vi "Post Substeps Digital Input Task.vi"(9 "Socket No":u16=1, 10 "DI In":T1, 11 "Sequence Context In":refnum<k7>) -> (0 "error out":errorcluster, 1 "PhysicalChannel":string[](array[string]), 2 "DigitalInputRead":bool[](array[boolean]), 3 "Report Text":string)   [LabVIEW 2023, in "LTT_TeststandSteptypes.lvlib"]
doc: "This VI is Anaload Input Read MultiNumeric Test and PostSub Steptypes"
uses:
  LTT_TeststandSteptypes.lvlib
  HardwareAbstractionLayer_LVOOP/Digital Input/DI_class/DI DAQ/Control/DI Step Control.ctl
  HardwareAbstractionLayer_LVOOP/Main/Class Options.ctl
  HardwareAbstractionLayer_LVOOP/Digital Input/DI_class/DI.lvclass
  HardwareAbstractionLayer_LVOOP/Main/Main.lvclass
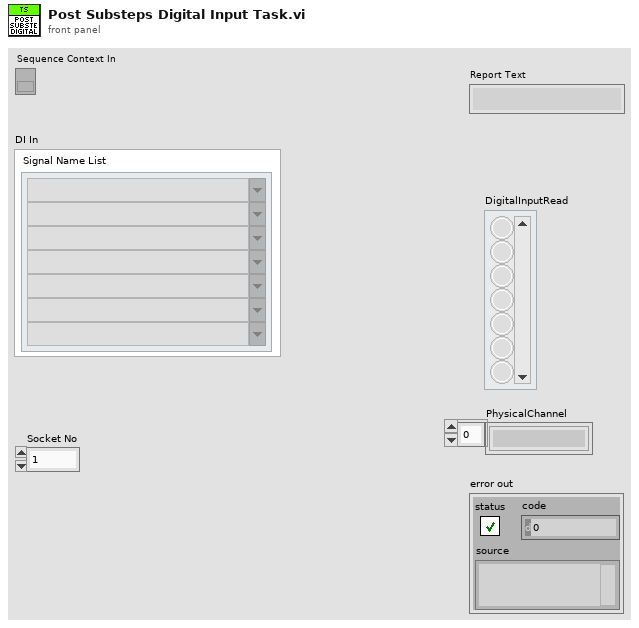
[diagram p1: front panel]
types:
  T1 = typedef "HardwareAbstractionLayer_LVOOP.lvlib/DI.lvclass/DI Step Control.ctl" = cluster{"Signal Name List":string[]}
  T2 = typedef "HardwareAbstractionLayer_LVOOP.lvlib/Main.lvclass/Class Options.ctl" = enum16{"Init All Class", "Read All Class", "Write AI Class", "Write AO Class", "Write AO Waveform Generation", "Write DI Class", "Write DO Class", "Write PWM Input Class", "Write PWM Output Class", "Exit"}
  T3 = typedef "HardwareAbstractionLayer_LVOOP.lvlib/Main.lvclass/Class Ref.ctl" = cluster{"FGV":refnum<class "Function Global Variable.lvclass">, "Notifier":refnum<class "NotifierHandler.lvclass">, "Queue":refnum<class "Queue Handler.lvclass">, "User Event":refnum<class "User Event.lvclass">, "Data Manager":refnum<class "Data Manager.lvclass">, "DMM":refnum<class "DMM.lvclass">, "Function Generator":refnum<class "Function Generator.lvclass">, "Oscilloscope":refnum<class "Oscilloscope.lvclass">, "PowerSupply":refnum<class "PowerSupply.lvclass">, "Teststand":refnum<class "Teststand.lvclass">, "AO":refnum<class "AO.lvclass">, "AI":refnum<class "AI.lvclass">, "Database":refnum<class "Database.lvclass">, "AO Waveform Generation":refnum<class "AO.lvclass">, "DO":refnum<class "DO.lvclass">, "DI":refnum<class "DI.lvclass">, "PWM Output":refnum<class "PWM Output.lvclass">, "PWM Input":refnum<class "PWM Input.lvclass">, "RelayOutput":refnum<class "NISwitch.lvclass">, "Modbus":refnum<class "Modbus.lvclass">, "CAN":refnum<class "CAN.lvclass">}
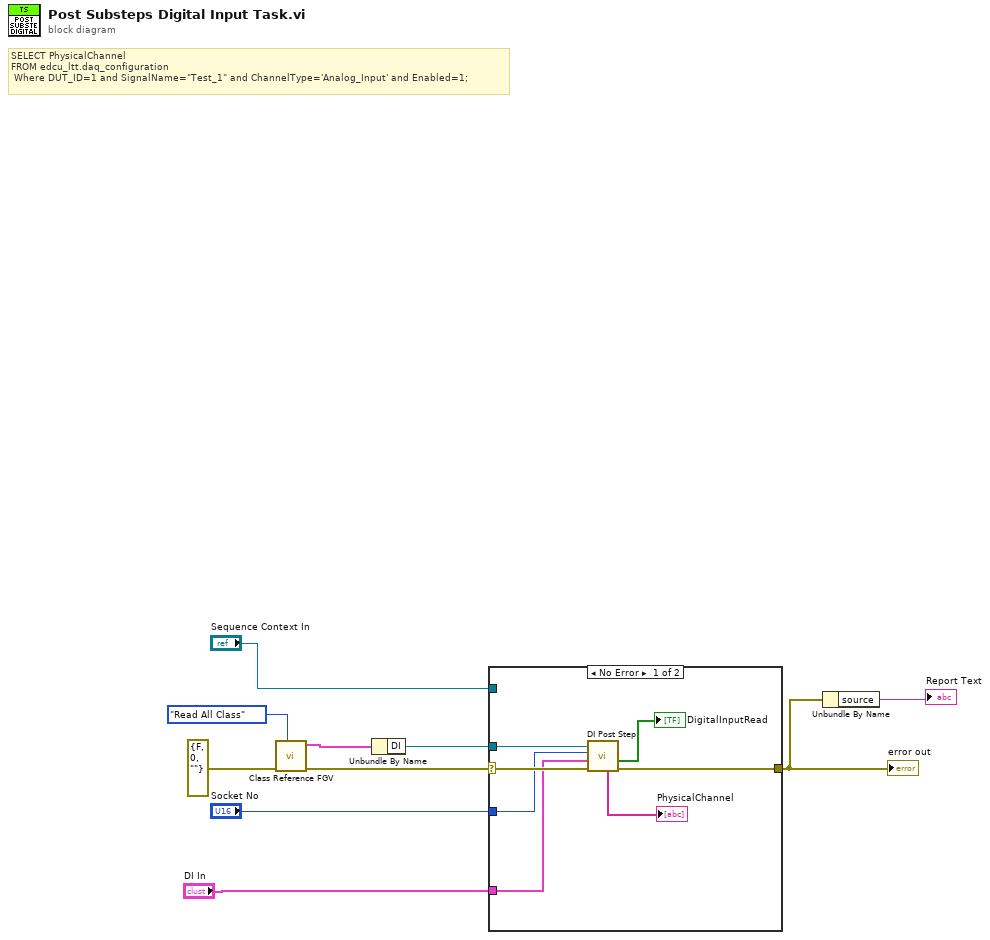
[diagram p0: block diagram]
diagram:
  # "SELECT PhysicalChannel \nFROM edcu_ltt.daq_configuration\n Where DUT_ID=1 and SignalName=\"Test_1\" and ChannelType='Analog_Input' and Enabled=1;"
  n1 = call "Class Reference FGV.vi"("Options"=Class_Options."Read All Class", "error in"=errorcluster {"status"=FALSE, "code"=0, "source"=""}) -> ("error out"=w7:errorcluster, "Class Cluster Out"=w9:T3)  [unwired: 8 in]
  n2 = Unbundle By Name(w9) -> ("DI"=w6:refnum<class "DI.lvclass">)
  n3 = case shown="No Error" w7 {
    selector: w7 -> [w16 w18]
    tunnel: w6 -> [w17 _]
    tunnel: [w15 w18] -> w5
    tunnel: "Socket No" -> [w13 _]
    tunnel: "DI In" -> [w12 _]
    tunnel: "Sequence Context In" -> [_ _]
    frame No Error {
      n4 = call-dynamic "DI Post Step.vi"("error in (no error)"=w16, "DI In"=w12, "Socket No"=w13, "DI in"=w17) -> ("error out"=w15:errorcluster, "DigitalRead"=→"DigitalInputRead":bool[], "PhysicalChannel"=→"PhysicalChannel":string[])  [unwired: 3 in, 2 out]
    }
    frame Error {
    }
  }
  "error out" <- w5
  n5 = Unbundle By Name(w5) -> ("source"=→"Report Text":string)
